vi "Waveform to FFT.vi"(8 "t < X ?":bool, 9 "Measured?":bool, 10 "Sampling Time(s)":i32, 11 "Waveform in":waveform(dbl)) -> (1 "FFT out":waveform(dbl), 2 "Last FFT":waveform(dbl), 3 "Last Waveform":waveform(dbl), 4 "Frequency":dbl)   [LabVIEW 2018]
uses:
  <vilib>/express/express analysis/Spectral/Block/exnSpectralBlock spectral measurements RMS poly.vi
  <vilib>/express/express analysis/Spectral/Block/exnSpectralBlock spectral measurements RMS WFM.vi
  <vilib>/express/express analysis/Spectral/XNode/ExpressSpectralMeasurementsBlockNode.xnode
panel:
  # "Inputs"
  # "Outputs"
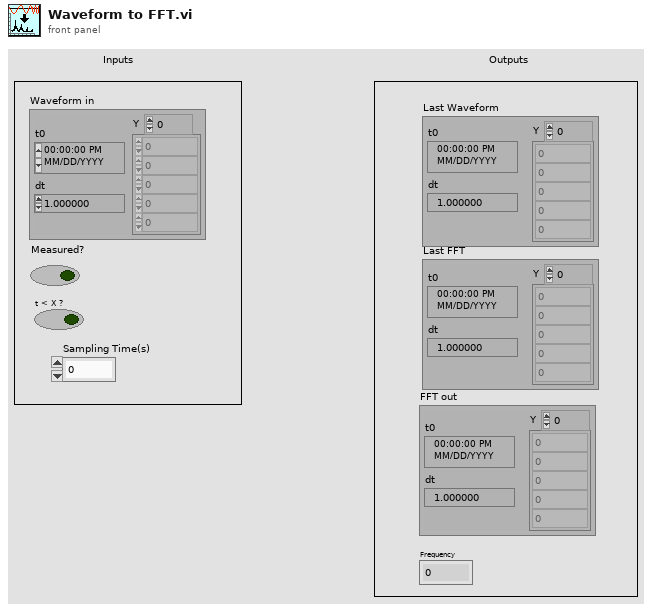
[diagram p1: front panel]
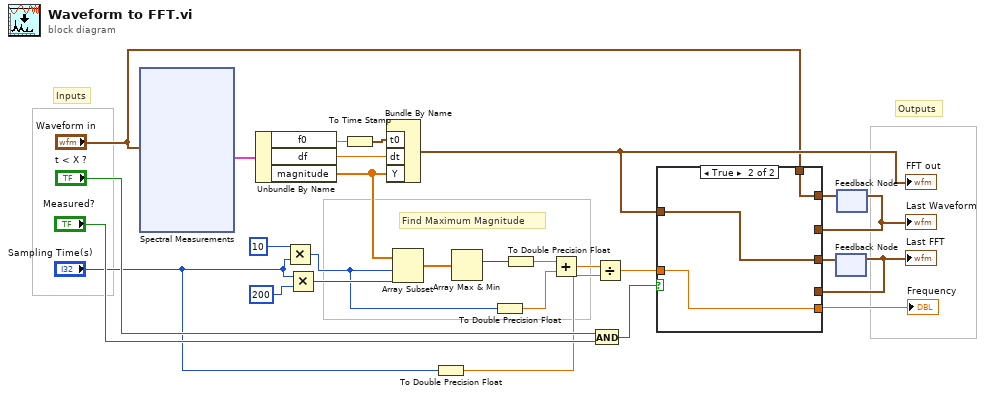
[diagram p0: block diagram]
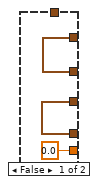
[diagram p2: hidden frame]
diagram:
  # "Outputs"
  # "Inputs"
  # "Find Maximum Magnitude"
  n1 = xnode "Spectral Measurements"("Signals"="Waveform in") -> ("FFT - (RMS)"=w23:cluster{"f0":dbl, "df":dbl, "magnitude":dbl[]})  [unwired: 1 in, 2 out]
  n2 = Unbundle By Name(w23) -> ("f0"=w21:dbl, "df"=w24:dbl, "magnitude"=w22:dbl[])
  n3 = Multiply(x=10, y="Sampling Time(s)") -> (x*y=w5:i32)
  n4 = Multiply(x="Sampling Time(s)", y=200) -> (x*y=w6:i32)
  n5 = To Time Stamp(1:w21) -> (0:w25:timestamp)
  n6 = Bundle By Name("t0"=w25, "dt"=w24, "Y"=w22) -> (w17:waveform(dbl))  [unwired: 1 in]
  "FFT out" <- w17
  n7 = Array Subset(array=w22, index=w5, length=w6) -> (w26:dbl[])
  n8 = To Double Precision Float(number="Sampling Time(s)") -> (double precision float=w2:dbl)
  n9 = Array Max & Min(array=w26) -> (max index (indices)=w20:i32)  [unwired: 3 out]
  n10 = To Double Precision Float(number=w5) -> (double precision float=w18:dbl)
  n11 = To Double Precision Float(number=w20) -> (double precision float=w19:dbl)
  n12 = Add(x=w19, y=w18) -> (x+y=w4:dbl)
  n13 = And(x="t < X ?", y="Measured?") -> (x .and. y?=w11:bool)
  n14 = Divide(x=w4, y=w2) -> (x/y=w3:dbl)
  n15 = feedback #1() -> (w14:waveform(dbl))  [unwired: 1 in]
  "Last FFT" <- w14
  n16 = feedback #2() -> (w12:waveform(dbl))  [unwired: 1 in]
  "Last Waveform" <- w12
  n17 = case shown="True" w11 {
    tunnel: w3 -> [_ w33]
    tunnel: [0.0 w33] -> w27
    tunnel: w17 -> [_ w32]
    tunnel: "Waveform in" -> [_ w31]
    tunnel: [w29 w32] -> w15
    tunnel: [w28 w31] -> w13
    tunnel: w14 -> [w29 _]
    tunnel: w12 -> [w28 _]
    frame False {
    }
    frame True {
    }
  }
  "Frequency" <- w27
  n18 = feedback-in #1(w15) -> ()
  n19 = feedback-in #2(w13) -> ()
